vi "Configure Setpoint.vi"(8 "error in (no error)":errorcluster, 10 "Setpoint Info In":T1={"Number"=0, "Enable"=FALSE, "Temperature"=0.0, "Window"=2.0, "Soak Time"=60, "Ramp Rate"=9999.0} {"Ramp Rate" min=0.0 max=9999.0 step=1.0 format="%.1f"; "Soak Time" min=0 max=9999 step=1 format="%#.0f"; "Window" min=0.1 max=9.9 step=0.1 format="%.1f"; "Temperature" min=-150.0 max=225.0 step=0.1 format="%.1f"; "Number" min=0 max=17}, 11 "VISA resource name":refnum<visa-resource-name>) -> (0 "error out":errorcluster, 3 "VISA resource name out":refnum<visa-resource-name>)   [LabVIEW 2012, in "Temptronic TP04300.lvlib"]
doc: "This VI allows to configure the setpoint parameters, such as\n\n<b>Setpoint Number</b>\nDefault Value: 0\nValid range: 0-17 - for the Cycle Screen\n 0-2 - for the Operator Screen\n \n<b>Setpoint Enable/disable</b> from the cycle list.\n0 - disable setpoint\n1 - enable setpoint\n\n<b>Setpoint temperature</b>\nValid Range: \n -150.0 to 225.0 in the Cycle Screen for any setpoint\n 25.0 to 225.0 for setpoint #0 in Operator Screen\n 15.0 to 35.0 for setpoint #1 in Operator Screen\n -150.0 to 25.0 for setpoint #2 in Operator Screen\n\nNote: Entering a value greater than maximum air temperature limit or\nless than minimum air temperature limit will cause \"out of range error\" \n\n\n<b>Setpoint temperature window</b>\nValid Range: 0.1 to 9.9 \nDefault Value: 2.0\n\nNote: The window is the maximum positive or negative deviation from \nthe temperature setpoint allowable for an \"at temperature\" condition. \n\n<b>Setpoint the soak time</b>\nValid Range: 0 to 9999\nDefault Value: 60\n\n<b>Setpoint ramp rate</b>\nValid Range: 0 to 99.9 with 0.1C temperature resolution\n or 100 to 9999 with 1C temperature resolution\nDefault Value: 9999"
uses:
  <instrlib>/Temptronic TP04300/Temptronic TP04300.lvlib
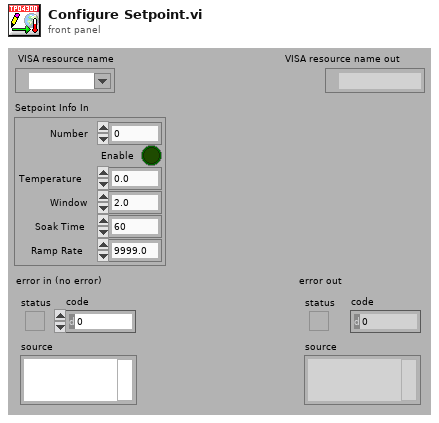
[diagram p1: front panel]
types:
  T1 = cluster{"Number":i32, "Enable":bool, "Temperature":dbl, "Window":dbl, "Soak Time":i32, "Ramp Rate":dbl}
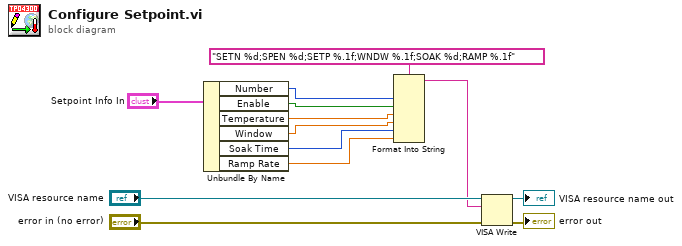
[diagram p0: block diagram]
diagram:
  n1 = Unbundle By Name("Setpoint Info In") -> ("Number"=w7:i32, "Enable"=w6:bool, "Temperature"=w2:dbl, "Window"=w1:dbl, "Soak Time"=w5:i32, "Ramp Rate"=w4:dbl)
  n2 = Format Into String(format string="SETN %d;SPEN %d;SETP %.1f;WNDW %.1f;SOAK %d;RAMP %.1f" ("multi-line string"), w7, w6, w2, w1, w5, w4) -> (resulting string=w9:string)  [unwired: 2 in, 1 out]
  n3 = VISA Write(VISA resource name="VISA resource name", write buffer=w9, error in (no error)="error in (no error)") -> (VISA resource name out=→"VISA resource name out":refnum<visa-resource-name>, error out=→"error out":errorcluster)  [unwired: 1 out]
